vi "Config Mngr.vi"(5 "Main References":T5, 7 "Mngr Action":T6, 8 "error in":errorcluster, 11 "path":path) -> (0 "error out":errorcluster, 1 "Config":T1={"Syringe size"=0, "Syringe address"=0, "# of ports"=0, "Init String"="Z0N1R", "Full Stroke (cnts)"=0, "Model"=enum."XC", "TW Position"=0.0, "Load Position"=0.0, "Bottom Position"=0.0, "Station ID"="", "Default Protocol"=path "", "Dry Time(s)"=0.0, "Python Version"="", "NFC SN Array"=["21121521200223", "21121521200186", "21121521200213", "52541737200062"], "Timing"={"Checking pres and leak"=0.0, "Priming input lines"=0.0, "Rinsing syringe"=0.0, "Filling well X w/ X"=0.0, "Drain well X"=0.0, "Clearing wells and lines"=0.0, "Draining wells"=0.0, "Rinsing all wells"=0.0, "Testing for leaks/clogs"=0.0, "Rinsing wells"=0.0}, "Pressure Specs"={"Pressure max"=0.0, "Pressure min"=0.0, "Decay delta"=0.0, "Pressure time"=0.0, "Conf. R"=0.0, "LeakRateMax"=0.0}}, 3 "path out":path)   [LabVIEW 2020]
uses:
  Config Mngr.ctl
  Main Refs.ctl
  Hardware/Tecan/Pump Config.ctl
  Timing Specs.ctl
  Vacuum Specs.ctl
  Cartridges.ctl
  Cartridge Status.ctl
  Commands.ctl
  Lib/Time/Wells.ctl
  Lib/Time/Bottles.ctl
  Process State.ctl
  Vacuum Test.ctl
  Wash Step.ctl
  Main Globals.vi
panel:
  out "Setup Array":T4[](array[typedef]) {"# of Rinses" max=10}
  # "Tecan Pump"
  # "Pressure"
  # "General"
  # "Timing"
  # "Protocol"
  # "Zaber"
  # "NFC Reader 1"
  # "NFC  Reader 2"
  # "NFC Reader 3"
  # "NFC Reader 4"
  # "Tecan Pump"
  # "Pressure"
  # "General"
  # "Timing"
  # "Protocol"
  # "Zaber"
  # "NFC Reader 1"
  # "NFC  Reader 2"
  # "NFC Reader 3"
  # "NFC Reader 4"
  # "System"
  # "Cartridge Utitlies"
  # "Wells"
  # "times"
  # "from"
  # "State Machine"
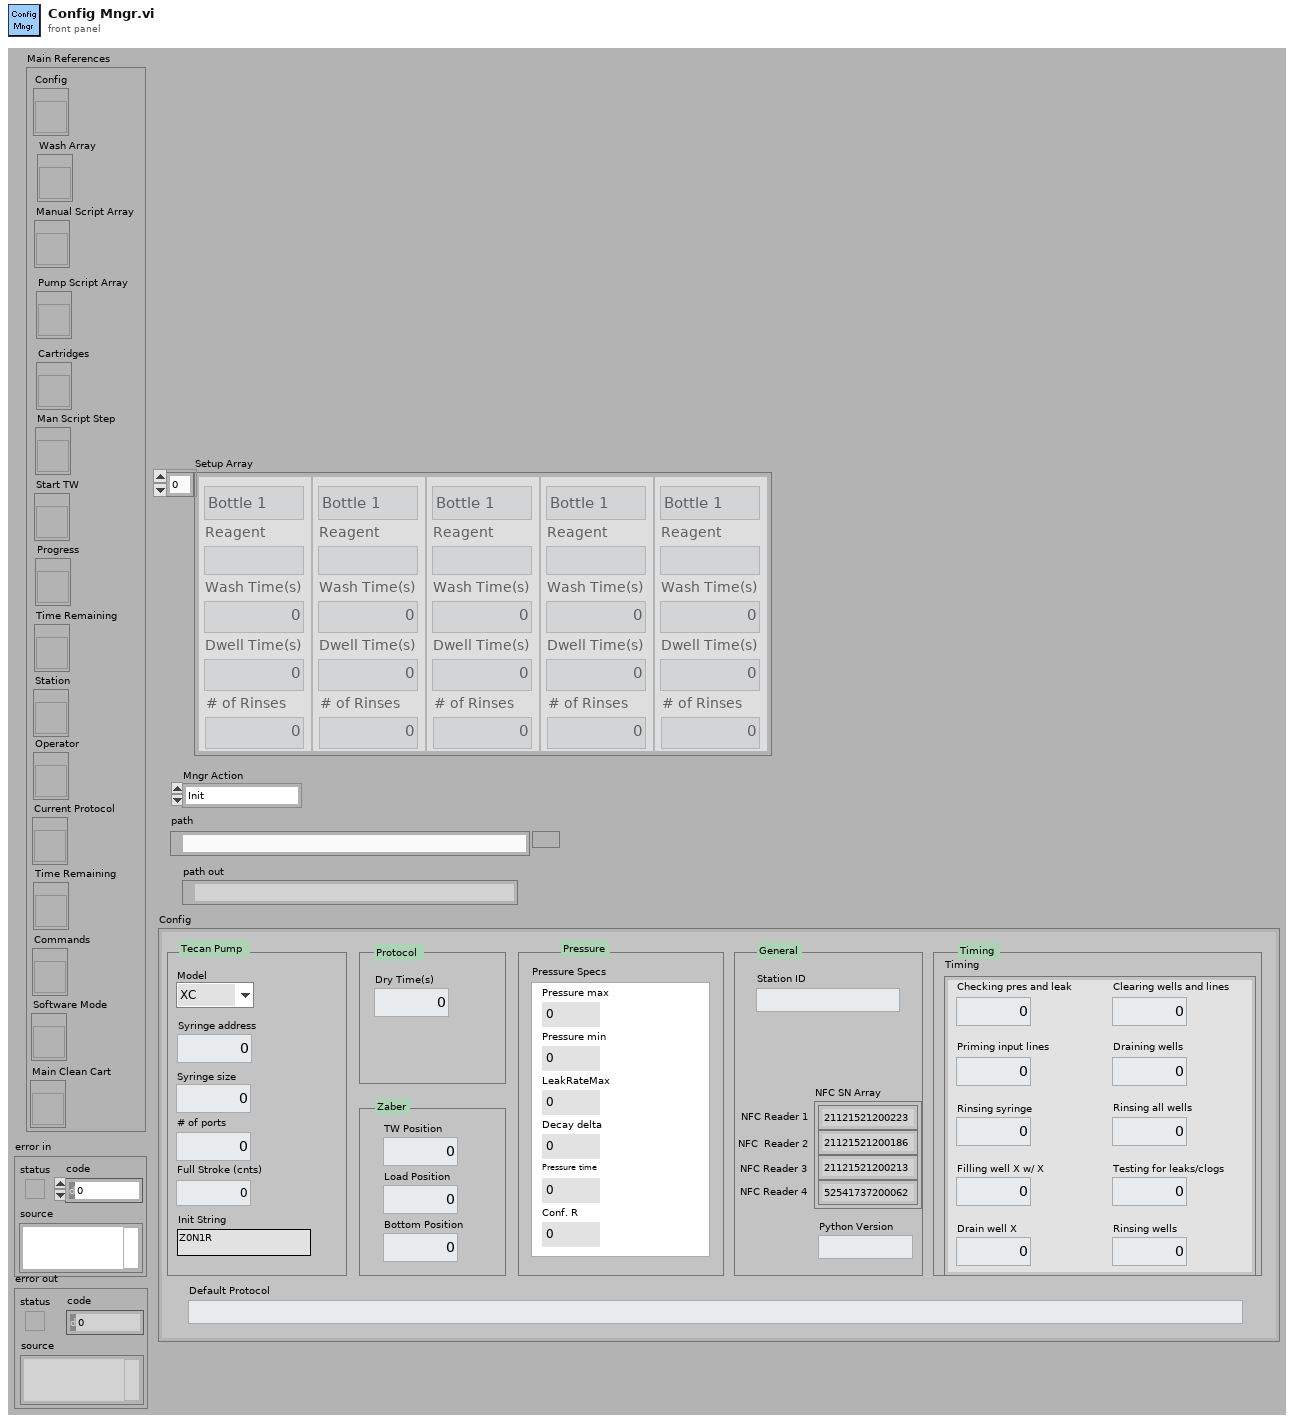
[diagram p1: front panel]
types:
  T1 = typedef "Pump Config.ctl" = cluster{"Syringe size":u32, "Syringe address":u32, "# of ports":u32, "Init String":string, "Full Stroke (cnts)":i32, "Model":enum16{"XC", "Centris"}, "TW Position":dbl, "Load Position":dbl, "Bottom Position":dbl, "Station ID":string, "Default Protocol":path, "Dry Time(s)":dbl, "Python Version":string, "NFC SN Array":string[], "Timing":T2, "Pressure Specs":T3}
  T2 = typedef "Timing Specs.ctl" = cluster{"Checking pres and leak":dbl, "Priming input lines":dbl, "Rinsing syringe":dbl, "Filling well X w/ X":dbl, "Drain well X":dbl, "Clearing wells and lines":dbl, "Draining wells":dbl, "Rinsing all wells":dbl, "Testing for leaks/clogs":dbl, "Rinsing wells":dbl}
  T3 = typedef "Vacuum Specs.ctl" = cluster{"Pressure max":dbl, "Pressure min":dbl, "Decay delta":dbl, "Pressure time":dbl, "Conf. R":dbl, "LeakRateMax":dbl}
  T4 = typedef "Wash Step.ctl" = cluster{"Reagent":string, "Bottle":enum16{"Bottle 1", "Bottle 2", "Bottle 3", "Bottle 4"}, "Wash Time(s)":dbl, "Dwell Time(s)":dbl, "# of Rinses":i16}
  T5 = typedef "Main Refs.ctl" = cluster{"Config":refnum<vi>, "Wash Array":refnum<vi>, "Manual Script Array":refnum<vi>, "Pump Script Array":refnum<vi>, "Cartridges":refnum<vi>, "Man Script Step":refnum<vi>, "Start TW":refnum<vi>, "Progress":refnum<vi>, "Time Remaining":refnum<vi>, "Station":refnum<vi>, "Operator":refnum<vi>, "Current Protocol":refnum<vi>, "Time Remaining":refnum<vi>, "Commands":refnum<vi>, "Software Mode":refnum<vi>, "Main Clean Cart":refnum<vi>}
  T6 = typedef "Config Mngr.ctl" = enum16{"Init", "Load Config", "Save Config", "Load Protocol", "Save Protocol", "Close"}
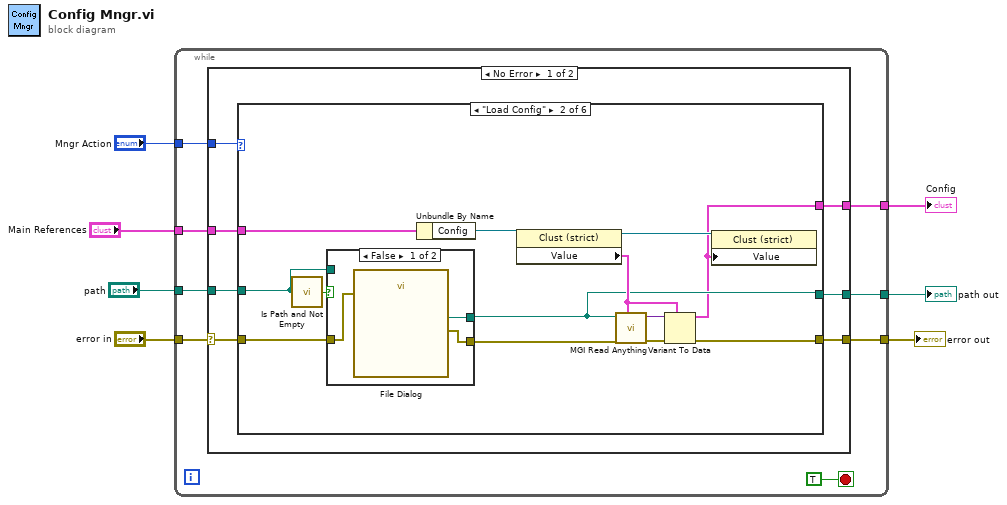
[diagram p0: block diagram]
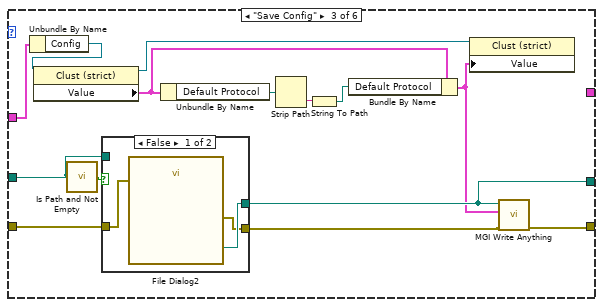
[diagram p4: hidden frame]
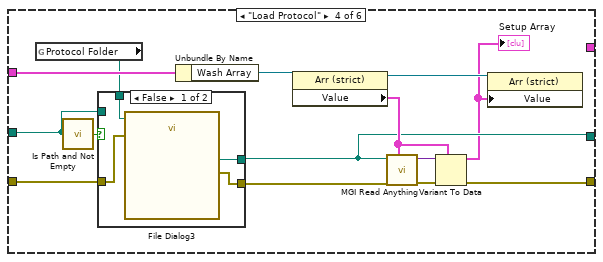
[diagram p6: hidden frame]
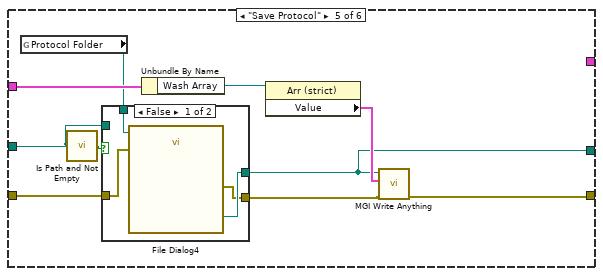
[diagram p8: hidden frame]
diagram:
  n1 = while {
    tunnel: "error in" -> [w11]
    tunnel: [w13] -> w6
    tunnel: "Mngr Action" -> [w14]
    tunnel: "Main References" -> [w12]
    tunnel: "path" -> [w10]
    tunnel: [w9] -> w3
    tunnel: [w8] -> w1
    stop <- TRUE stop-if-true
    n2 = case shown="No Error" w11 {
      selector: w11 -> [w19 w99]
      tunnel: w14 -> [w22 _]
      tunnel: [w21 w99] -> w13
      tunnel: w12 -> [w20 _]
      tunnel: w10 -> [w18 w98]
      tunnel: [w17 w98] -> w9
      tunnel: [w16 _] -> w8
      frame No Error {
        n3 = case shown="\"Load Config\"" w22 {
          tunnel: w19 -> [w23 w27 w52 w65 w85 w97]
          tunnel: [w23 w35 w54 w73 w89 w97] -> w21
          tunnel: w20 -> [_ w36 w55 w74 w90 _]
          tunnel: w18 -> [_ w28 w50 w66 w83 _]
          tunnel: [_ w25 w49 w63 w82 _] -> w17
          tunnel: [_ w24 _ _ _ _] -> w16
          frame "Init" {
          }
          frame "Load Config" {
            n4 = call <vilib>:"Is Path and Not Empty.vi"("path"=w28) -> ("Is Path and Not Empty?"=w29:bool)  [unwired: 4 in]
            n5 = case shown="False" w29 {
              tunnel: [w39 w41] -> w25
              tunnel: w28 -> [_ w41]
              tunnel: w27 -> [w38 w40]
              tunnel: [w37 w40] -> w26
              frame False {
                n6 = call "File Dialog"("error in"=w38) -> ("selected path"=w39:path, "error out"=w37:errorcluster)  [unwired: 11 in, 2 out]
              }
              frame True {
              }
            }
            n7 = Unbundle By Name(w36) -> ("Config"=w34:refnum<vi>)
            n8 = property class="Clust (strict)"(reference=w34) -> (reference out=w33:refnum<vi>, "Value"=w30:T1)  [unwired: 1 in, 1 out]
            n9 = call <userlib>:"MGI Read Anything.vi"("Type of Anything"=w30, "Error In"=w26, "Path (dialog)"=w25) -> ("Error Out"=w32:errorcluster, "Anything"=w31:variant)  [unwired: 5 in, 2 out]
            n10 = Variant To Data(error in=w32, type=w30, Variant=w31) -> (data=w24:T1, error out=w35:errorcluster)
            n11 = property class="Clust (strict)"(reference=w33, "Value"=w24) -> ()  [unwired: 1 in, 2 out]
          }
          frame "Save Config" {
            n12 = Unbundle By Name(w55) -> ("Config"=w46:refnum<vi>)
            n13 = property class="Clust (strict)"(reference=w46) -> (reference out=w43:refnum<vi>, "Value"=w47:T1)  [unwired: 1 in, 1 out]
            n14 = call <vilib>:"Is Path and Not Empty.vi"("path"=w50) -> ("Is Path and Not Empty?"=w53:bool)  [unwired: 4 in]
            n15 = case shown="False" w53 {
              tunnel: [w58 w60] -> w49
              tunnel: w50 -> [_ w60]
              tunnel: w52 -> [w57 w59]
              tunnel: [w56 w59] -> w51
              frame False {
                n16 = call "File Dialog2"("error in"=w57) -> ("selected path"=w58:path, "error out"=w56:errorcluster)  [unwired: 11 in, 2 out]
              }
              frame True {
              }
            }
            n17 = Unbundle By Name(w47) -> ("Default Protocol"=w48:path)
            n18 = Strip Path(path=w48) -> (name=w45:string)  [unwired: 1 out]
            n19 = String To Path(string=w45) -> (path=w44:path)
            n20 = Bundle By Name(cluster=w47, "Default Protocol"=w44) -> (w42:T1)
            n21 = property class="Clust (strict)"(reference=w43, "Value"=w42) -> ()  [unwired: 1 in, 2 out]
            n22 = call <userlib>:"MGI Write Anything.vi"("Error In"=w51, "Anything"=w42, "Path (dialog)"=w49) -> ("Error Out"=w54:errorcluster)  [unwired: 6 in, 2 out]
          }
          frame "Load Protocol" {
            n23 = global read "Main Globals.vi" "Protocol Folder"() -> (w61:path)
            n24 = call <vilib>:"Is Path and Not Empty.vi"("path"=w66) -> ("Is Path and Not Empty?"=w67:bool)  [unwired: 4 in]
            n25 = case shown="False" w67 {
              tunnel: [w78 w80] -> w63
              tunnel: w66 -> [_ w80]
              tunnel: w65 -> [w77 w79]
              tunnel: [w76 w79] -> w64
              tunnel: w61 -> [w75 _]
              frame False {
                n26 = call "File Dialog3"("start path"=w75, "error in"=w77) -> ("selected path"=w78:path, "error out"=w76:errorcluster)  [unwired: 10 in, 2 out]
              }
              frame True {
              }
            }
            n27 = Unbundle By Name(w74) -> ("Wash Array"=w72:refnum<vi>)
            n28 = property class="Arr (strict)"(reference=w72) -> (reference out=w71:refnum<vi>, "Value"=w68:T4[])  [unwired: 1 in, 1 out]
            n29 = call <userlib>:"MGI Read Anything.vi"("Type of Anything"=w68, "Error In"=w64, "Path (dialog)"=w63) -> ("Error Out"=w70:errorcluster, "Anything"=w69:variant)  [unwired: 5 in, 2 out]
            n30 = Variant To Data(error in=w70, type=w68, Variant=w69) -> (data=w62:T4[], error out=w73:errorcluster)
            "Setup Array" <- w62
            n31 = property class="Arr (strict)"(reference=w71, "Value"=w62) -> ()  [unwired: 1 in, 2 out]
          }
          frame "Save Protocol" {
            n32 = global read "Main Globals.vi" "Protocol Folder"() -> (w81:path)
            n33 = call <vilib>:"Is Path and Not Empty.vi"("path"=w83) -> ("Is Path and Not Empty?"=w86:bool)  [unwired: 4 in]
            n34 = case shown="False" w86 {
              tunnel: [w94 w96] -> w82
              tunnel: w83 -> [_ w96]
              tunnel: w85 -> [w93 w95]
              tunnel: [w92 w95] -> w84
              tunnel: w81 -> [w91 _]
              frame False {
                n35 = call "File Dialog4"("start path"=w91, "error in"=w93) -> ("selected path"=w94:path, "error out"=w92:errorcluster)  [unwired: 10 in, 2 out]
              }
              frame True {
              }
            }
            n36 = Unbundle By Name(w90) -> ("Wash Array"=w88:refnum<vi>)
            n37 = property class="Arr (strict)"(reference=w88) -> ("Value"=w87:T4[])  [unwired: 1 in, 2 out]
            n38 = call <userlib>:"MGI Write Anything.vi"("Error In"=w84, "Anything"=w87, "Path (dialog)"=w82) -> ("Error Out"=w89:errorcluster)  [unwired: 6 in, 2 out]
          }
          frame "Close" {
          }
        }
      }
      frame Error {
      }
    }
  }
  "error out" <- w6
  "path out" <- w3
  "Config" <- w1
